vi "instToJson.vi"(11 "instruction type":T1) -> (3 "instruction template":string)   [LabVIEW 2017]
uses:
  list-commands-names.ctl
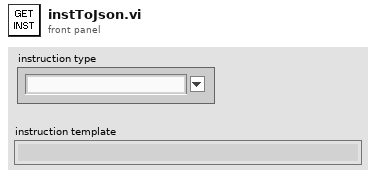
[diagram p1: front panel]
types:
  T1 = typedef "list-commands-names.ctl" = string
  T2 = cluster{"label":string, "inst":string, "seconds":dbl}
  T3 = cluster{"label":string, "inst":string, "next-label":string, "maxcounts":dbl}
  T4 = cluster{"label":string, "inst":string, "filename":string}
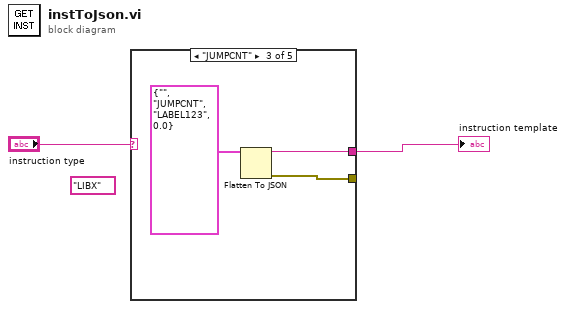
[diagram p0: block diagram]
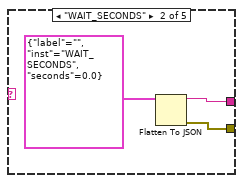
[diagram p3: hidden frame]
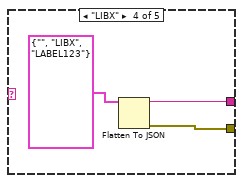
[diagram p4: hidden frame]
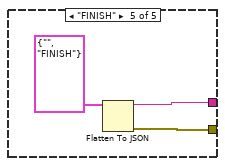
[diagram p5: hidden frame]
diagram:
  (unwired) T1 "LIBX" ("instruction")
  n1 = case shown="\"JUMPCNT\"" "instruction type" {
    tunnel: [_ w5 w7 w10 w14] -> w2
    tunnel: [_ w4 w6 w9 w13] -> _
    frame Default {
    }
    frame "WAIT_SECONDS" {
      n2 = Flatten To JSON(anything=T2 {"label"="", "inst"="WAIT_SECONDS", "seconds"=0.0} ("Cluster")) -> (JSON string=w5:string, 11:w4:errorcluster)  [unwired: 2 in]
    }
    frame "JUMPCNT" {
      n3 = Flatten To JSON(anything=T3 {"label"="", "inst"="JUMPCNT", "next-label"="LABEL123", "maxcounts"=0.0} ("Cluster")) -> (JSON string=w7:string, 11:w6:errorcluster)  [unwired: 2 in]
    }
    frame "LIBX" {
      n4 = Flatten To JSON(anything=T4 {"label"="", "inst"="LIBX", "filename"="LABEL123"} ("Cluster")) -> (JSON string=w10:string, 11:w9:errorcluster)  [unwired: 2 in]
    }
    frame "FINISH" {
      n5 = Flatten To JSON(anything=cluster{"label":string, "inst":string} {"label"="", "inst"="FINISH"} ("Cluster")) -> (JSON string=w14:string, 11:w13:errorcluster)  [unwired: 2 in]
    }
  }
  "instruction template" <- w2
